vi "Append to Buffer.vi"(8 "error in":errorcluster, 10 "Channel":string, 11 "BufferLastReadingsDBL in":refnum<class "BufferLastReadsDBL.lvclass">) -> (0 "error out":errorcluster, 3 "BufferLastReadingsDBL out":refnum<class "BufferLastReadsDBL.lvclass">)   [LabVIEW 2024, in "BufferLastReadsDBL.lvclass"]
uses:
  BufferLastReadsDBL.lvclass
  BufferLastReadsDBL.lvclass/BufferLastReadsDBL.ctl
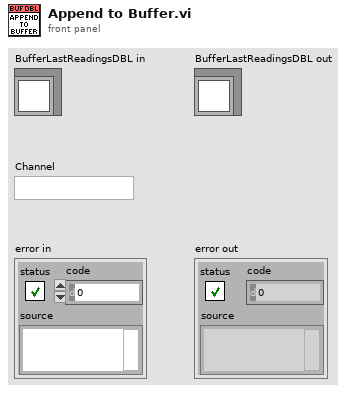
[diagram p1: front panel]
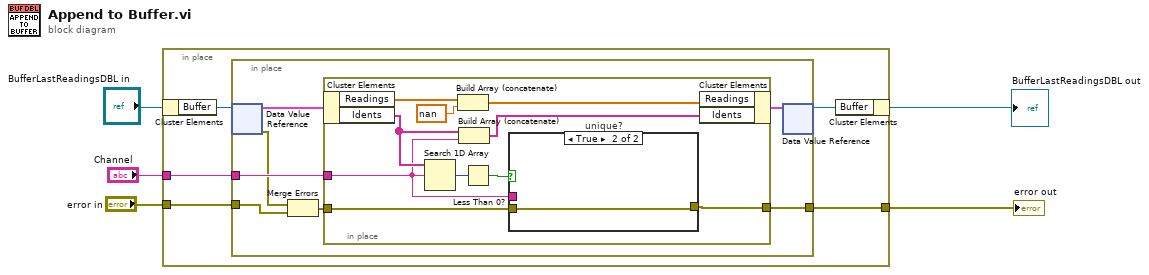
[diagram p0: block diagram]
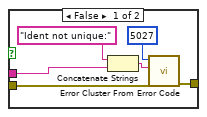
[diagram p2: hidden frame]
diagram:
  n1 = in-place {
    in-place-border: "Channel" -> [w8]
    in-place-border: "error in" -> [w7]
    in-place-border: [w6] -> w1
    n2 = in-place-cluster #1("BufferLastReadingsDBL in") -> ("Buffer"=w10:refnum<data-value>)
    n3 = in-place {
      in-place-border: w8 -> [w16]
      in-place-border: w7 -> [w14]
      in-place-border: [w17] -> w6
      n4 = in-place-dvr #2(w10) -> (w12:cluster{"Idents":string[], "Readings":dbl[]}, w13:errorcluster)
      n5 = Merge Errors(w13, w14) -> (w15:errorcluster)
      n6 = in-place {
        in-place-border: [w25] -> w17
        in-place-border: w16 -> [w18]
        in-place-border: w15 -> [w24]
        n7 = in-place-cluster #3(w12) -> ("Readings"=w23:dbl[], "Idents"=w21:string[])
        n8 = Search 1D Array(1D array=w21, element=w18) -> (index of element=w26:i32)  [unwired: 1 in]
        n9 = Build Array (concatenate)(w23, nan) -> (w20:dbl[])
        n10 = Build Array (concatenate)(w21, w18) -> (w19:string[])
        n11 = Less Than 0?(x=w26) -> (x < 0?=w27:bool)
        n12 = case "unique?" shown="True" w27 {
          tunnel: w24 -> [w33 w34]
          tunnel: [w32 w34] -> w25
          tunnel: w18 -> [w28 _]
          frame False {
            n13 = Concatenate Strings("Ident not unique:" ("string"), w28) -> (w30:string)
            n14 = call <vilib>:"Error Cluster From Error Code.vi"("error in (no error)"=w33, "error message (\"\")"=w30, "error code (0)"=5027) -> ("error out"=w32:errorcluster)  [unwired: 6 in]
          }
          frame True {
          }
        }
        n15 = in-place-cluster #3("Readings"=w20, "Idents"=w19) -> (w11:cluster{"Idents":string[], "Readings":dbl[]})
      }
      n16 = in-place-dvr #2(w11) -> (w9:refnum<data-value>)  [unwired: 1 out]
    }
    n17 = in-place-cluster #1("Buffer"=w9) -> (→"BufferLastReadingsDBL out":refnum<class "BufferLastReadsDBL.lvclass">)
  }
  "error out" <- w1
